vi "Configure TCP Connection.vi"(4 "Read Mode (Immediate)":T1(ring)=enum."Immediate", 6 "timeout (5000ms)":i32=5000, 8 "error in (no error)":errorcluster, 10 "remote port (80)":u16=80, 11 "address (localhost)":string="localhost") -> (0 "error out":errorcluster, 3 "TCPConnection":refnum<class "TCPConnection.lvclass">)   [LabVIEW 2013, in "MQTT_TCP.lvlib" / "TCPConnection.lvclass"]
uses:
  TCPConnection.lvclass
  TCPConnection.lvclass/TCPConnection.ctl
  <vilib>/LabVIEW Open Source Project/MQTT Connection/MQTT_Connection/Connection/Connection.lvclass/Connection.ctl
  <vilib>/LabVIEW Open Source Project/MQTT Connection/MQTT_Connection/Connection/Connection.lvclass
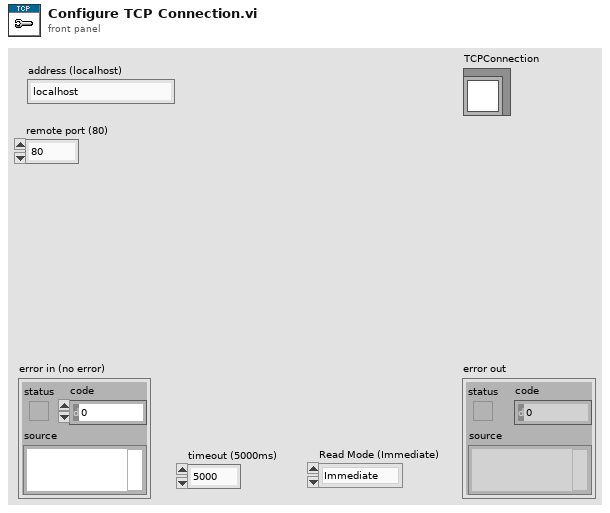
[diagram p1: front panel]
types:
  T1 = enum16{"Standard", "Buffered", "CRLF", "Immediate"}
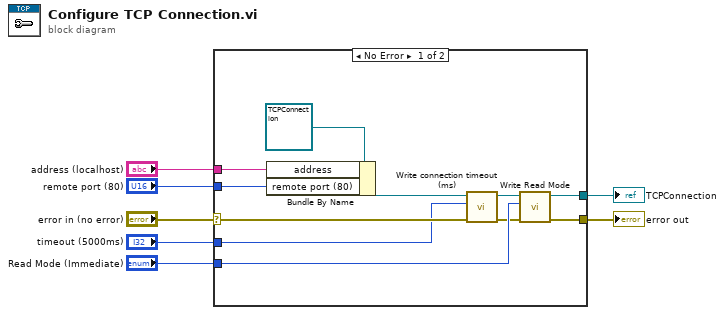
[diagram p0: block diagram]
diagram:
  n1 = case shown="No Error" "error in (no error)" {
    selector: "error in (no error)" -> [w14 w19]
    tunnel: [w8 w19] -> w6
    tunnel: [w10 _] -> w2
    tunnel: "address (localhost)" -> [w17 _]
    tunnel: "remote port (80)" -> [w16 _]
    tunnel: "timeout (5000ms)" -> [w13 _]
    tunnel: "Read Mode (Immediate)" -> [w12 _]
    frame No Error {
      n2 = Bundle By Name(cluster=refnum<class "TCPConnection.lvclass"> refnum ("TCPConnection in"), "address"=w17, "remote port (80)"=w16) -> (w15:refnum<class "TCPConnection.lvclass">)
      n3 = call <vilib>:"Write connection timeout (ms).vi"("error in (no error)"=w14, "connection timeout (ms)"=w13, "Connection in"=w15) -> ("error out"=w9:errorcluster, "Connection out"=w11:refnum<class "TCPConnection.lvclass">)  [unwired: 7 in]
      n4 = call "Write Read Mode.vi"("error in (no error)"=w9, "Read Mode"=w12, "TCPConnection in"=w11) -> ("error out"=w8:errorcluster, "TCPConnection"=w10:refnum<class "TCPConnection.lvclass">)  [unwired: 7 in]
    }
    frame Error {
    }
  }
  "error out" <- w6
  "TCPConnection" <- w2
